vi "AddNumericArrays.vi"(9 "Array 2":dbl[](array[numeric]), 11 "Array":dbl[](array[numeric])) -> (3 "Sum":dbl[](array[numeric]))   [LabVIEW 2012]
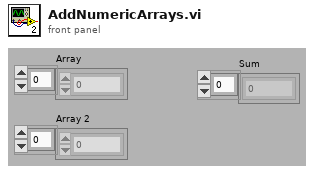
[diagram p1: front panel]
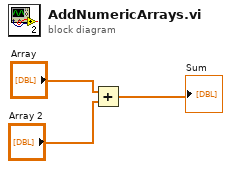
[diagram p0: block diagram]
diagram:
  n1 = Add(x="Array", y="Array 2") -> (x+y=→"Sum":dbl[])
